vi "PID.vi"(6 "previous (in)":cluster{"error":dbl, "integral":dbl}={"error"=inf, "integral"=inf}, 7 "range":cluster{"max":dbl, "min":dbl}={"max"=100.0, "min"=-100.0}, 8 "coeffecients":cluster{"P":dbl, "I":dbl, "D":dbl}={"P"=1.0, "I"=0.0, "D"=0.0}, 9 "time":dbl, 10 "process variable":dbl, 11 "setpoint":dbl) -> (2 "output":dbl, 4 "previous (out)":cluster{"error":dbl, "integral":dbl})   [LabVIEW 2009]
panel:
  # "P  I  D"
  # "http://en.wikipedia.org/wiki/PID_controller"
  # "This VI is compatible with the LabVIEW NXT toolkit 2.0"
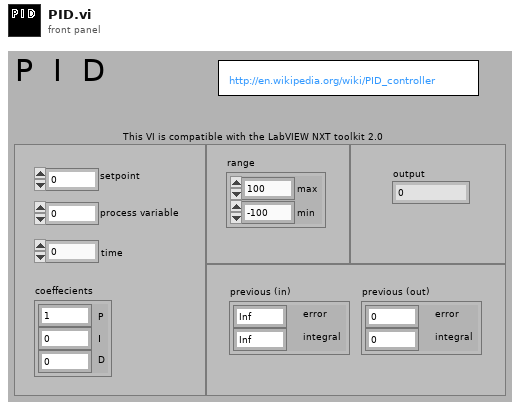
[diagram p1: front panel]
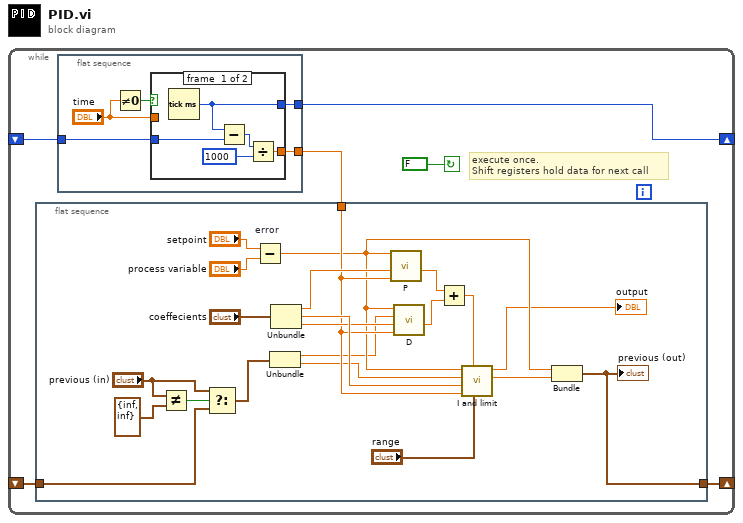
[diagram p0: block diagram]
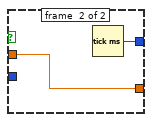
[diagram p2: hidden frame]
diagram:
  n1 = while {
    shift-right: [w4] -> _
    shift-left: _ -> [w5]
    shift-right: [w1] -> _
    shift-left: _ -> [w2]
    stop <- FALSE continue-if-true
    # "execute once.\nShift registers hold data for next call"
    n2 = flat-sequence {
      tunnel: w3 -> [w25]
      tunnel: w2 -> [w20]
      tunnel: [w19] -> w1
      frame #0 {
        n3 = Not Equal?(x="previous (in)", y=cluster{"error":dbl, "integral":dbl} {"error"=inf, "integral"=inf} ("previous")) -> (x != y?=w23:bool)
        n4 = Select(t="previous (in)", s=w23, f=w20) -> (s? t:f=w21:cluster{"error":dbl, "integrated error":dbl})
        n5 = Subtract "error"(x="setpoint", y="process variable") -> (x-y=w16:dbl)
        n6 = Unbundle(w21) -> ("error"=w14:dbl, "integrated error"=w13:dbl)
        n7 = Unbundle("coeffecients") -> ("P"=w28:dbl, "I"=w27:dbl, "D"=w26:dbl)
        n8 = call "P.vi"("change time"=w25, "P gain"=w28, "error"=w16) -> ("output"=w12:dbl)  [unwired: 8 in]
        n9 = call "D.vi"("change time"=w25, "D gain"=w26, "prev error"=w14, "error"=w16) -> ("output"=w11:dbl)  [unwired: 7 in]
        n10 = Add(x=w12, y=w11) -> (x+y=w10:dbl)
        n11 = call "I and limit.vi"("range"="range", "P + D outputs"=w10, "change time"=w25, "I gain"=w27, "integrated error"=w13, "error"=w16) -> ("integrated error"=w8:dbl, "output"=→"output":dbl)  [unwired: 3 in, 1 out]
        n12 = Bundle(w16, "integrated error"=w8) -> (w19:cluster{dbl, "integrated error":dbl})  [unwired: 1 in]
        "previous (out)" <- w19
      }
    }
    n13 = flat-sequence {
      tunnel: w5 -> [w33]
      tunnel: [w32] -> w4
      tunnel: [w31] -> w3
      frame #0 {
        n14 = Not Equal To 0?(x="time") -> (x != 0?=w30:bool)
        n15 = case shown="True" w30 {
          tunnel: w33 -> [w38 _]
          tunnel: [w37 w39] -> w32
          tunnel: [w34 w40] -> w31
          tunnel: "time" -> [_ w40]
          frame #0 {
            n16 = Tick Count (ms)() -> (millisecond timer value=w37:u32)
            n17 = Subtract(x=w37, y=w38) -> (x-y=w36:u32)
            n18 = Divide(x=w36, y=u32 1000) -> (x/y=w34:dbl)
          }
          frame #1 {
            n19 = Tick Count (ms)() -> (millisecond timer value=w39:u32)
          }
        }
      }
    }
  }
